vi "test_cleanup.vi"   [LabVIEW 2020]
uses:
  <instrlib>/AIM GmbH/_AIM 664/AIM664LV.lvlib
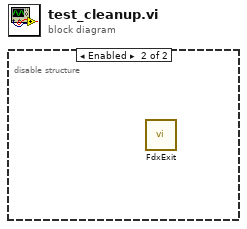
[diagram p0: block diagram]
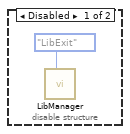
[diagram p2: hidden frame]
diagram:
  n1 = disable-structure shown="Enabled" {
    frame Disabled {
      n2 = call <instrlib>:"LibManager.vi"("action"=enum16{"LibInit", "LibExit"}."LibExit") -> ()  [unwired: 8 in, 3 out]
    }
    frame Enabled {
      n3 = call <instrlib>:"FdxExit.vi"() -> ()  [unwired: 11 in, 1 out]
    }
  }
